vi "Run Dual Mode Thermometer XControl.vi"(11 "Dual Mode Thermometer\nControl (DMTC)":dbl(xcontrol)=28.09917355371901) -> ()   [LabVIEW 2013]
doc: "This VI demonstrates the functionality of the Dual Mode Thermometer XControl. \n\nUsing different combinations of the mode on the DMTC and the DMTI will demonstrate the Dual Mode Thermometer XControl's functionality. The Fahrenheit Mode? boolean is indicating whether the DMTI is in Fahrenheit mode by using a custom Property created for the DMT XControl. The Converter converts Celcius to Fahrenheit using a Convert C to F method created for the DMT XControl. Refer to the Project Explorer and the XControl Help for more information on XControls."
uses:
  Simple Dual Mode Thermometer XControl.xctl
panel:
  out "Degrees Fahrenheit":dbl
  in  "Degrees Celsius":dbl
  out "Fahrenheit?":bool
  out "Dual Mode Thermometer\nIndicator (DMTI)":dbl(xcontrol)=28.09917355371901
  in  "stop":bool
  # "Operating Instructions:\n\n1. Run the VI\n2. Adjust the DMTC\n3. Select the Fahrenheit mode of DMTC\n4. Adjust the DMTC\n5. Select the Fahrenheit mode of DMTI\n6. Adjust the DMTC\n7. Stop the VI\n\nUsing different combinations of the mode on the DMTC and the DMTI will demonstrate the Dual Mode Thermometer XControl's functionality. \n\nThe Fahrenheit Mode? boolean is indicating whether the DMTI is in Fahrenheit mode by using a custom Property created for the DMT XControl. \n\nThe  Converter converts Celsius to Fahrenheit using a Convert C to F method created for the DMT XControl.  \n\nRefer to the Project Explorer and the XControl Help for more information on XControls."
  # "NOTE: Close this VI before attempting to\nmake any changes to the Dual Mode\nThermometer XControl"
  # "Temperature Converter"
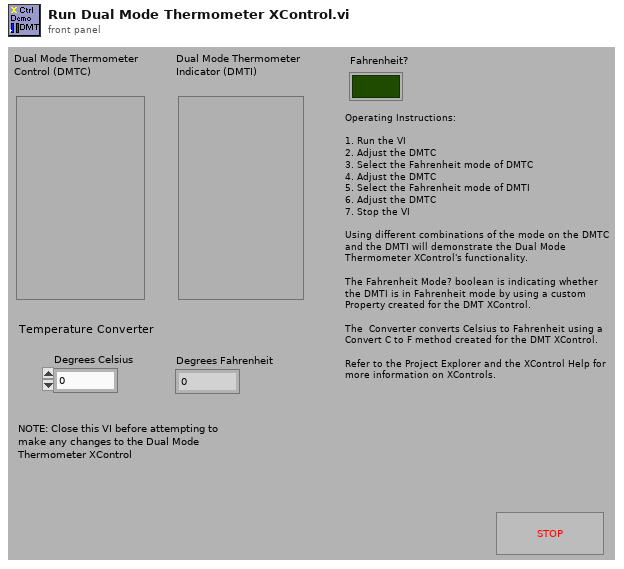
[diagram p1: front panel]
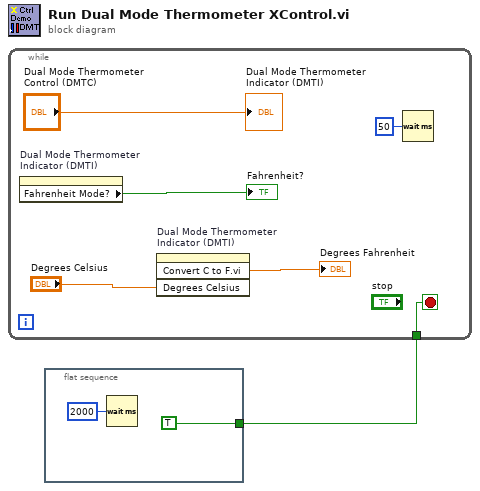
[diagram p0: block diagram]
diagram:
  n1 = while {
    tunnel: w1 -> [w2]
    stop <- w2 stop-if-true
    n2 = property on="Dual Mode Thermometer\nIndicator (DMTI)" class="Simple Dual Mode Thermometer XC"() -> ("Fahrenheit Mode?"=→"Fahrenheit?":bool)  [unwired: 2 in, 2 out]
    n3 = invoke on="Dual Mode Thermometer\nIndicator (DMTI)" class="Simple Dual Mode Thermometer XC" method="Convert C to F.vi"("Degrees Celsius"="Degrees Celsius") -> ("Convert C to F.vi"=→"Degrees Fahrenheit":dbl)  [unwired: 3 in, 3 out]
    n4 = Wait (ms)(milliseconds to wait=u32 50) -> ()  [unwired: 1 out]
    "Dual Mode Thermometer\nIndicator (DMTI)" <- "Dual Mode Thermometer\nControl (DMTC)"
  }
  n5 = flat-sequence {
    tunnel: [TRUE ("stop")] -> w1
    frame #0 {
      n6 = Wait (ms)(milliseconds to wait=u32 2000) -> ()  [unwired: 1 out]
    }
  }
